vi "filter_load_xml.vi"(8 "error in":errorcluster) -> (0 "error out":errorcluster, 3 "Filter Cluster":T1)   [LabVIEW 2013]
uses:
  filters.ctl
  <vilib>/Utility/xml.llb/Read From XML File(string).vi
panel:
  in  "Filter Cluster example":T1
  # "Regions of Interest -->"
  # "Shots\n   |\n  V"
  # "Counters -->"
  # "Counter\n    bins\n       |\n      V"
  # "Regions of Interest -->"
  # "Shots\n   |\n  V"
  # "Counters -->"
  # "Counter\n    bins\n       |\n      V"
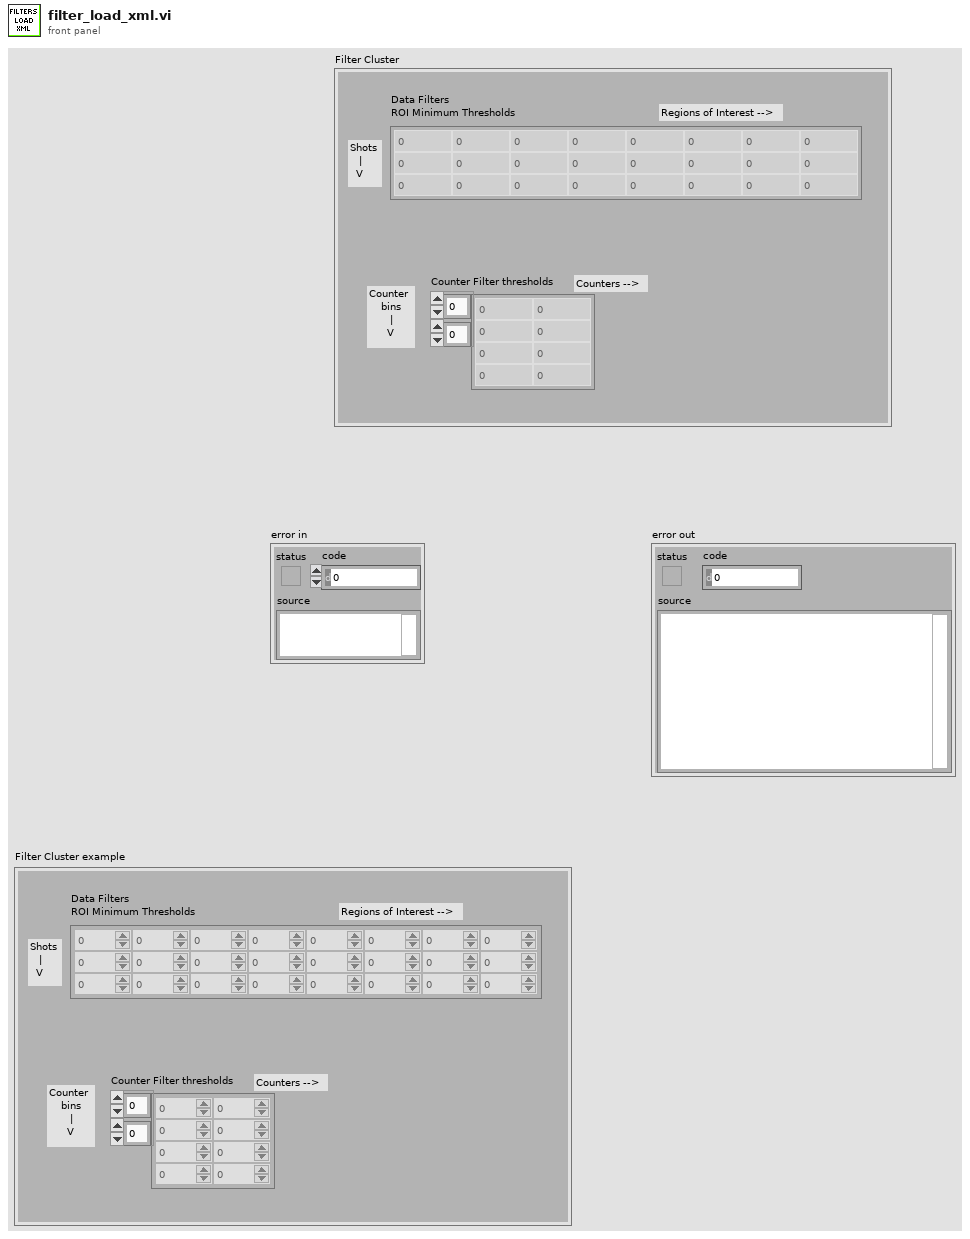
[diagram p1: front panel]
types:
  T1 = typedef "filters.ctl" = cluster{"Counter Filter thresholds":u32[][], "Data Filters\nROI Minimum Thresholds":u64[][]}
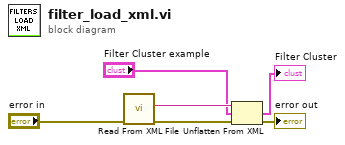
[diagram p0: block diagram]
diagram:
  n1 = call-poly <vilib>:"Read From XML File.vi"("error in (no error)"="error in") -> ("error out"=w4:errorcluster, "XML Elements"=w5:string)  [unwired: 8 in, 1 out]
  n2 = Unflatten From XML(xml string=w5, type="Filter Cluster example", error in (no error)=w4) -> (value=→"Filter Cluster":T1, error out=→"error out":errorcluster)
